vi "Etalon Position Plotter.vi"() -> ()   [LabVIEW 2010]
panel:
  out "XY Graph of Etalon Positions":cluster{dbl, dbl}[](graph)
  out "Loop Counter":i32
  in  "Stop":bool
  out "Thin Etalon Position":dbl
  out "Thick Etalon Position":dbl
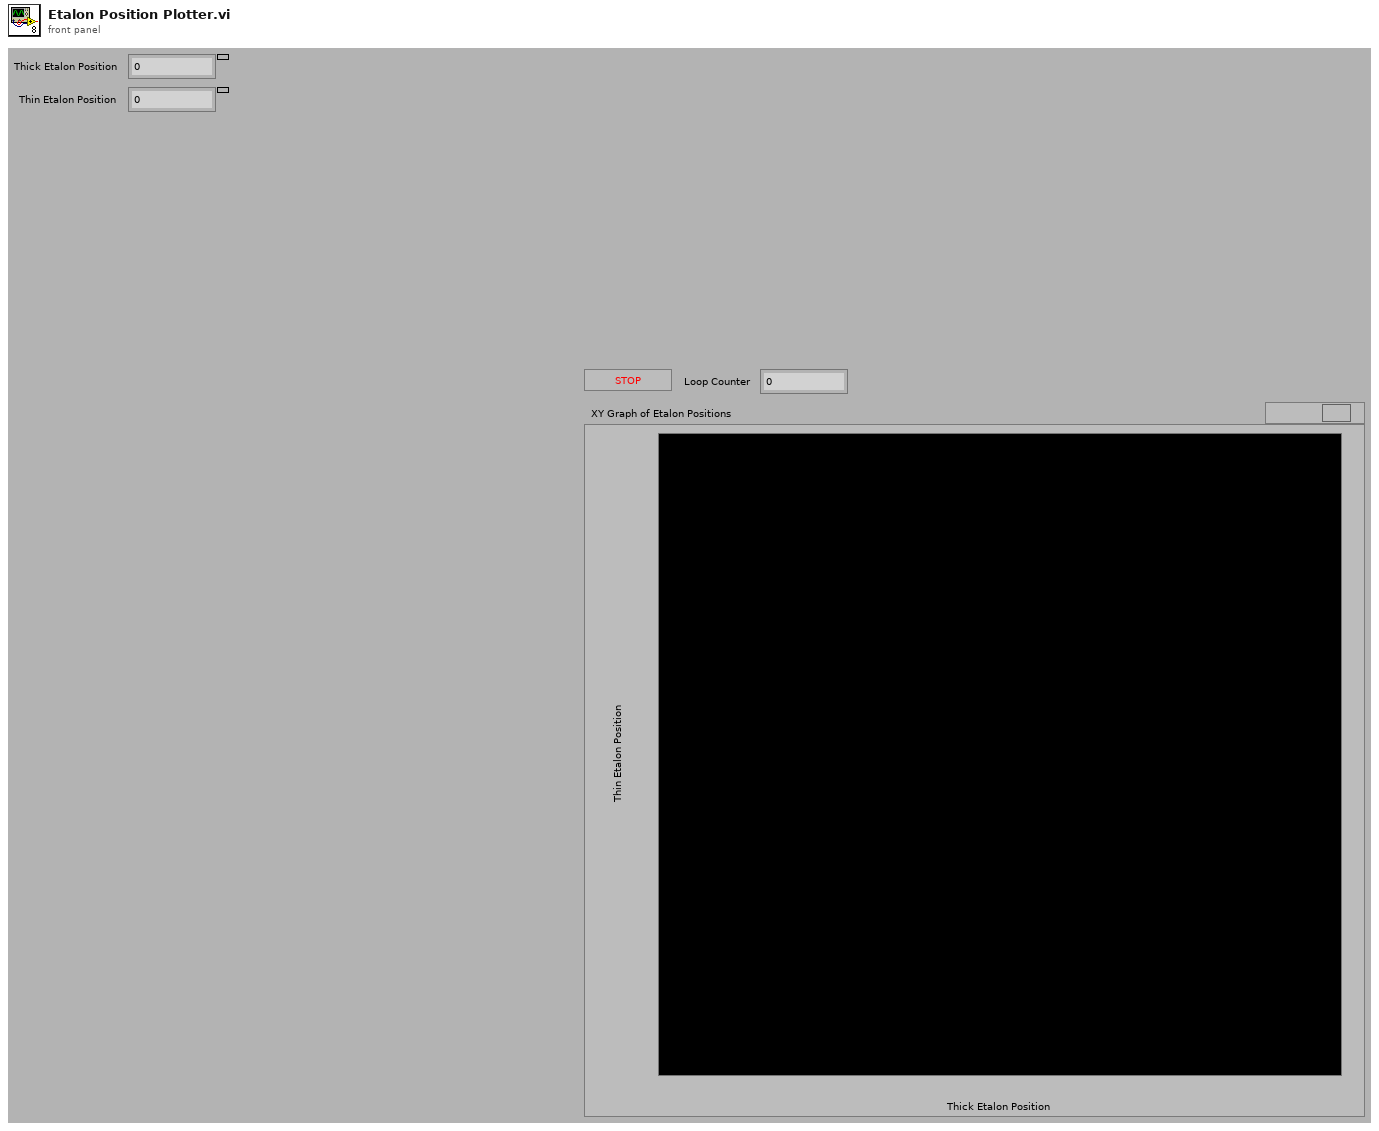
[diagram p1: front panel]
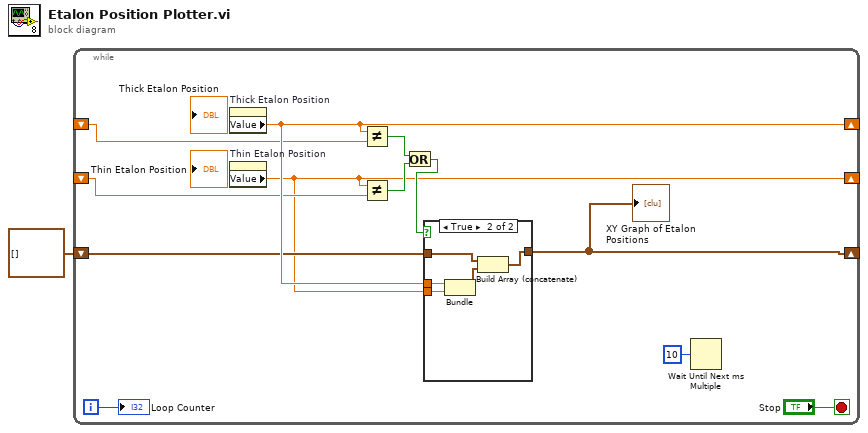
[diagram p0: block diagram]
diagram:
  n1 = while {
    shift-right: [w4] -> _
    shift-left: cluster{"Value":dbl, "Value":dbl}[] [] -> [w5]
    shift-right: [w11] -> _
    shift-left: _ -> [w10]
    shift-right: [w2] -> _
    shift-left: _ -> [w9]
    i -> [w12]
    stop <- "Stop" stop-if-true
    n2 = property on="Thick Etalon Position" class="DigNum (strict)"() -> ("Value"=w11:dbl)  [unwired: 2 in, 2 out]
    n3 = property on="Thin Etalon Position" class="DigNum (strict)"() -> ("Value"=w2:dbl)  [unwired: 2 in, 2 out]
    n4 = Not Equal?(x=w11, y=w10) -> (x != y?=w8:bool)
    n5 = Not Equal?(x=w2, y=w9) -> (x != y?=w7:bool)
    n6 = Or(x=w8, y=w7) -> (x .or. y?=w6:bool)
    n7 = case shown="True" w6 {
      tunnel: w11 -> [_ w19]
      tunnel: w2 -> [_ w18]
      tunnel: [w14 w16] -> w4
      tunnel: w5 -> [w14 w15]
      frame False {
      }
      frame True {
        n8 = Bundle("Value"=w19, "Value"=w18) -> (w17:cluster{"Value":dbl, "Value":dbl})  [unwired: 1 in]
        n9 = Build Array (concatenate)(w15, w17) -> (w16:cluster{"Value":dbl, "Value":dbl}[])
      }
    }
    "XY Graph of Etalon Positions" <- w4
    n10 = Wait Until Next ms Multiple(millisecond multiple=u32 10) -> ()  [unwired: 1 out]
    "Loop Counter" <- w12
  }
